vi "Actor Core.vi"(8 "error in":errorcluster, 11 "CS++PPGGUI.lvclass":refnum<class "CS++PPGGui.lvclass">) -> (0 "Error Out":errorcluster, 3 "Actor out":refnum<class "Actor.lvclass">)   [LabVIEW 2016, in "CS++PPGGui.lvlib" / "CS++PPGGui.lvclass"]
doc: "(<B>Filename</B>: Actor Framework.lvlib:Actor.lvclass:Actor Core.vi)\n\nReceives messages to the actor, reacts to them, and initiates any error handling that may shut the actor down.\n\nDescendant classes may override this VI to append parallel tasks for the actor to complete while it handles messages. Overrides use the Call Parent Method node."
uses:
  CS++PPGGui.lvclass
  CSPP_Core/Actors/CS++BaseActor/CS++BaseActor.lvclass
  <vilib>/ActorFramework/Actor/Actor.lvclass
  <vilib>/ActorFramework/Stop Msg/Stop Msg.lvclass
  CSPP_Core/Classes/CS++ProcessVariables/PVConnection/PVConnection.lvclass
  <vilib>/ActorFramework/Message Enqueuer/Message Enqueuer.lvclass
  CSPP_Core/Actors/CS++GUIActor/CS++GUIActor.lvclass
  CSPP_Core/Classes/CS++ProcessVariables/ProcessVariable/PV.lvclass
  CSPP_Core/Actors/CS++DeviceGUIActor/CS++DeviceGUIActor.lvclass
  CSPP_Core/Libraries/Utilities/CS++Utilities.lvlib
  C:/User/Brand/LVP/CSPP-Dev/Packages/CSPP_Core/Actors/CS++DeviceGUIActor/CS++DeviceGUIActor.lvclass
  C:/User/Brand/LVP/CSPP-Dev/Packages/CSPP_Core/Actors/CS++GUIActor/CS++GUIActor.lvclass
  C:/User/Brand/LVP/CSPP-Dev/Packages/CSPP_Core/Actors/CS++BaseActor/CS++BaseActor.lvclass
  C:/Program Files (x86)/National Instruments/LabVIEW 2016/vi.lib/ActorFramework/Actor/Actor.lvclass
panel:
  in  "Tab Control":enum32{"Info", "Control"}(tab)
  out "Last Update":timestamp
  out "Associated Device Actor":string
  out "Resource Name":string
  out "Self-Test Result Message":string
  out "Self-Test Result Code":i32
  out "Firmware Revision":string
  out "Driver Revision":string
  in  "Output":i32(listbox)
  in  "Ext Trig Button":bool
  in  "Abort Button":bool
  in  "Start Single Button":bool
  out "Status String":string
  in  "Pattern2FPGA Button":bool
  in  "Save Button":bool
  in  "Load Button":bool
  out "Error String":string
  in  "Stop Button":bool
  in  "Start Button":bool
  in  "Timing":i32(listbox)
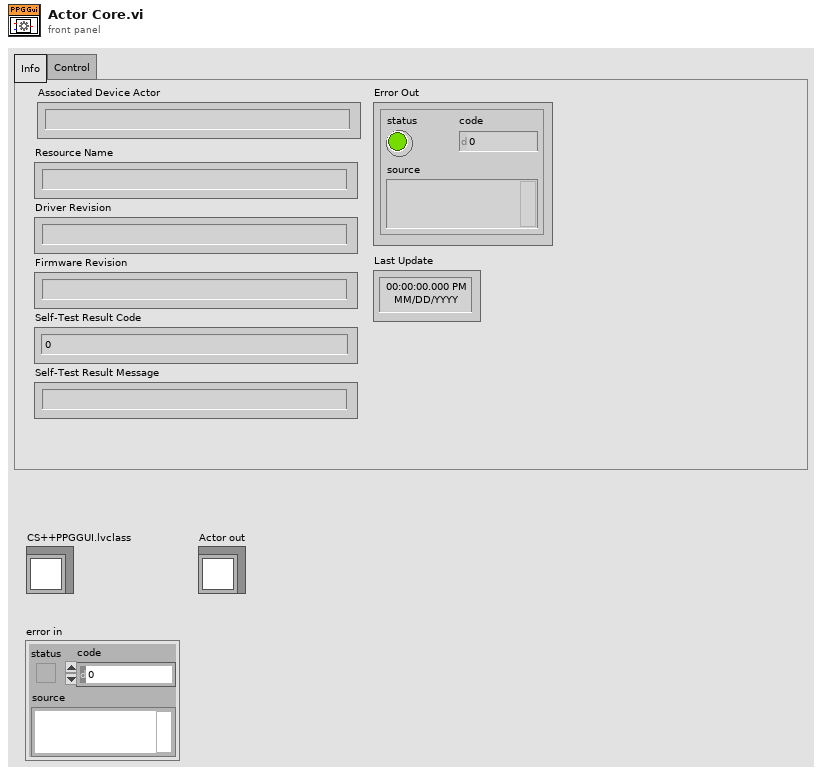
[diagram p1: front panel]
types:
  T1 = enum32{"Invalid", "Standard", "Closed", "Hidden", "Minimized", "Maximized"}
  T2 = enum16{"open", "replace", "create", "open or create", "replace or create", "replace or create with confirmation"}
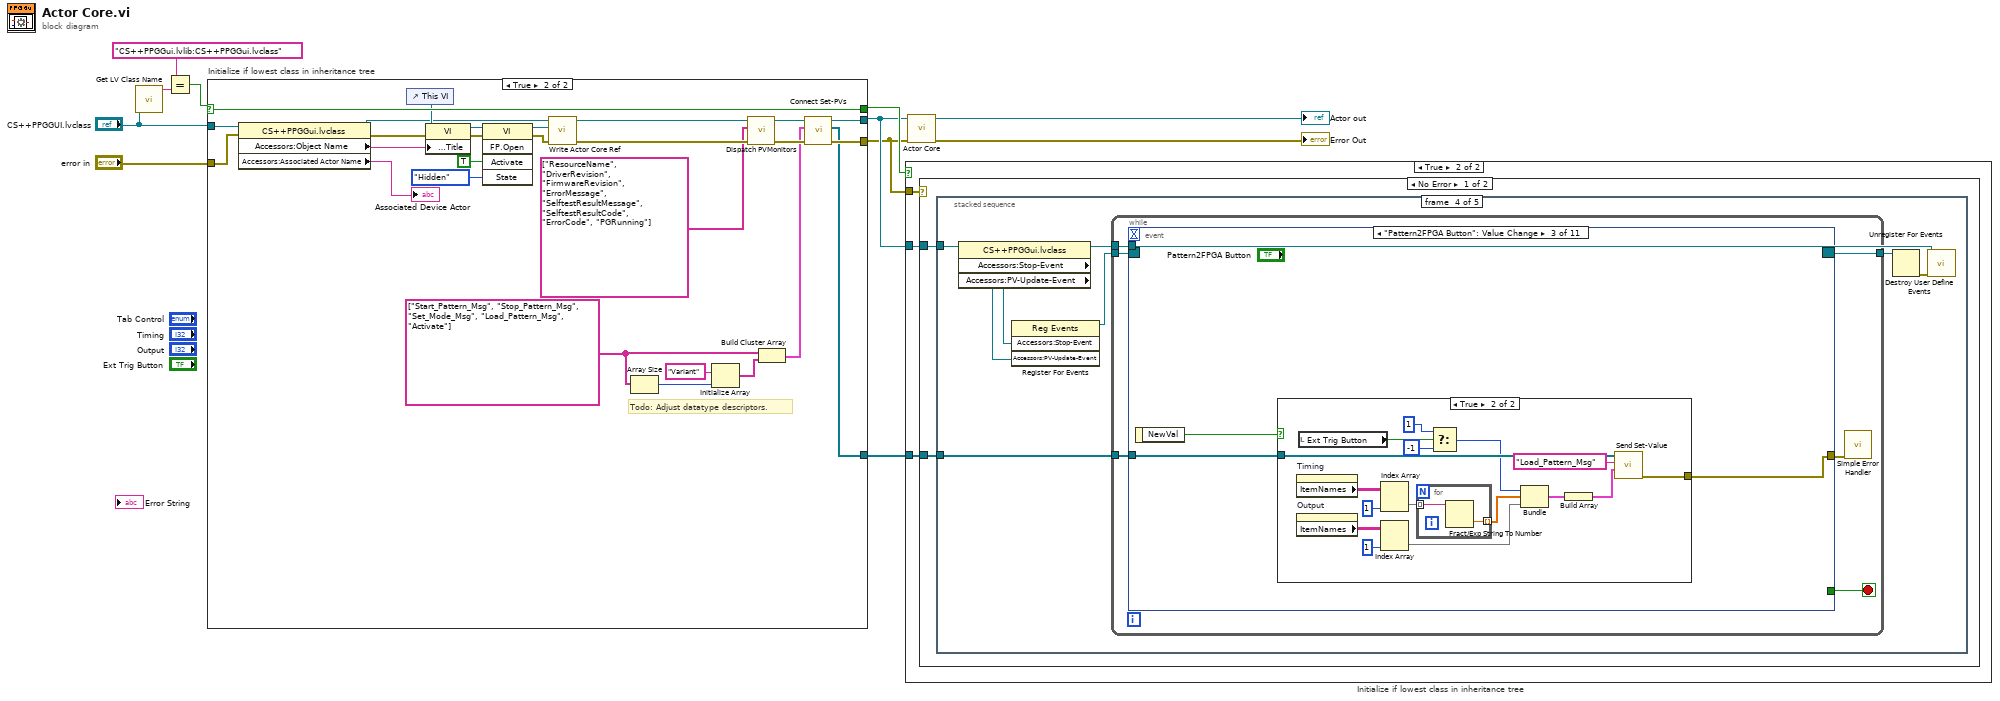
[diagram p0: block diagram]
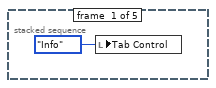
[diagram p4: hidden frame]
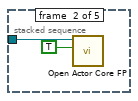
[diagram p5: hidden frame]
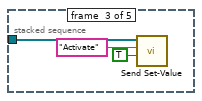
[diagram p6: hidden frame]
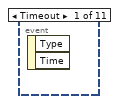
[diagram p7: hidden frame]
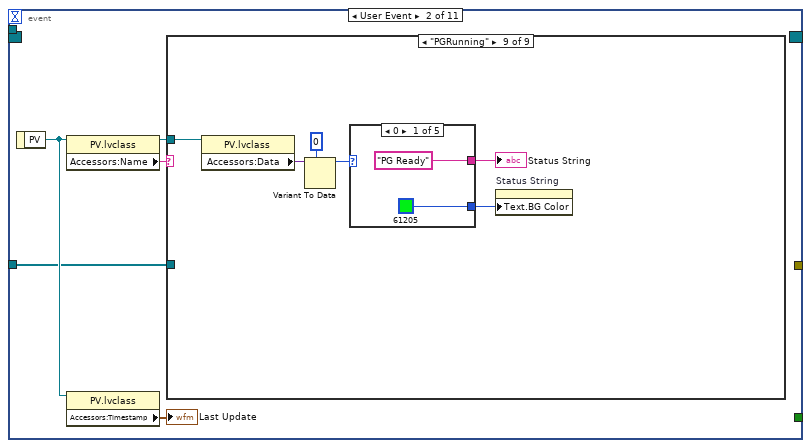
[diagram p8: hidden frame]
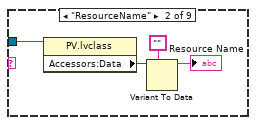
[diagram p10: hidden frame]
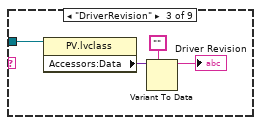
[diagram p11: hidden frame]
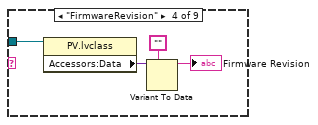
[diagram p12: hidden frame]
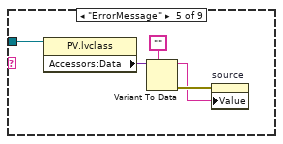
[diagram p13: hidden frame]
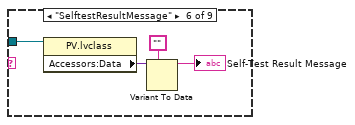
[diagram p14: hidden frame]
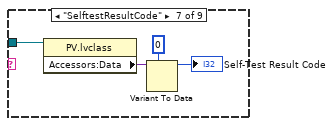
[diagram p15: hidden frame]
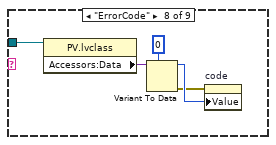
[diagram p16: hidden frame]
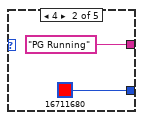
[diagram p17: hidden frame]
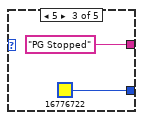
[diagram p18: hidden frame]
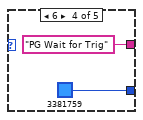
[diagram p19: hidden frame]
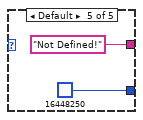
[diagram p20: hidden frame]
diagram:
  n1 = call <vilib>:"Get LV Class Name.vi"("object"="CS++PPGGUI.lvclass") -> ("class name"=w11:string)  [unwired: 9 in, 1 out]
  n2 = Equal?(x="CS++PPGGui.lvlib:CS++PPGGui.lvclass" ("class name"), y=w11) -> (x = y?=w9:bool)
  n3 = case "Initialize if lowest class in inheritance tree" shown="True" w9 {
    selector: w9 -> [w12 w41]
    tunnel: [w13 w24] -> w6
    tunnel: "error in" -> [w13 w28]
    tunnel: [w14 w25] -> w7
    tunnel: "CS++PPGGUI.lvclass" -> [w14 w29]
    tunnel: [w12 w41] -> w8
    tunnel: [_ w22] -> w5
    frame False {
    }
    frame True {
      w21 = string[] ["Start_Pattern_Msg", "Stop_Pattern_Msg", "Set_Mode_Msg", "Load_Pattern_Msg", "Activate"]
      # "Todo: Adjust datatype descriptors."
      n4 = property class="CS++PPGGui.lvclass"(reference=w29, error in=w28) -> (reference out=w33:refnum<class "CS++PPGGui.lvclass">, error out=w27:errorcluster, "Accessors:Object Name"=w32:string, "Accessors:Associated Actor Name"=→"Associated Device Actor":string)
      n5 = control-ref of="This VI"() -> (w36:refnum<vi>)
      n6 = property class="VI"(reference=w36, error in=w27, "Front Panel.Title"=w32) -> (reference out=w35:refnum<vi>, error out=w34:errorcluster)
      n7 = invoke class="VI" method="FP.Open"(reference=w35, error in=w34, "Activate"=TRUE ("Activate?"), "State"=T1."Hidden") -> (reference out=w38:refnum<vi>, error out=w37:errorcluster)  [unwired: 1 in, 3 out]
      n8 = call "Write Actor Core Ref.vi"("error in (no error)"=w37, "Actor Core Ref"=w38, "CS++BaseActor in"=w33) -> ("error out"=w30:errorcluster, "CS++BaseActor out"=w31:refnum<class "CS++PPGGui.lvclass">)  [unwired: 7 in]
      n9 = Array Size(array=w21) -> (size(s)=w20:i32)
      n10 = Initialize Array("Variant", w20) -> (w17:string[])
      n11 = call "Dispatch PVMonitors.vi"("Error In"=w30, "PV Names (empty)"=string[] ["ResourceName", "DriverRevision", "FirmwareRevision", "ErrorMessage", "SelftestResultMessage", "SelftestResultCode", "ErrorCode", "PGRunning"], "CS++GUIActor in"=w31) -> ("Error Out"=w23:errorcluster, "CS++GUIActor out"=w26:refnum<class "CS++PPGGui.lvclass">)  [unwired: 7 in]
      n12 = Build Cluster Array(w21, w17) -> (w18:cluster{string, string}[])
      n13 = call "Connect Set-PVs.vi"("Error In"=w23, "Set-Messages"=w18, "CS++GUIActor in"=w26) -> ("Error Out"=w24:errorcluster, "PVConnections"=w22:refnum<class "PVConnection.lvclass">[], "CS++GUIActor out"=w25:refnum<class "CS++PPGGui.lvclass">)  [unwired: 6 in]
    }
  }
  n14 = case "Initialize if lowest class in inheritance tree" shown="True" w8 {
    tunnel: w6 -> [_ w44]
    tunnel: w7 -> [_ w43]
    tunnel: w5 -> [_ w42]
    frame False {
    }
    frame True {
      n15 = case shown="No Error" w44 {
        tunnel: w43 -> [w46 _]
        tunnel: w42 -> [w45 _]
        frame No Error {
          n16 = stacked-sequence {
            tunnel: w46 -> [_ w48 _ w58 w271]
            tunnel: w45 -> [_ _ w50 w53 w269]
            frame #0 {
              n17 = local write "Tab Control"(enum32{"Info", "Control"}."Info" ("Tab Control")) -> ()
            }
            frame #1 {
              n18 = call "Open Actor Core FP.vi"("Open FP (F)"=TRUE, "CS++BaseActor in"=w48) -> ()  [unwired: 8 in, 2 out]
            }
            frame #2 {
              n19 = call "Send Set-Value.vi"("Data"=TRUE, "PVName"="Activate", "PVConnections"=w50) -> ()  [unwired: 7 in, 2 out]
            }
            frame #3 {
              n20 = property class="CS++PPGGui.lvclass"(reference=w58) -> (reference out=w57:refnum<class "CS++PPGGui.lvclass">, "Accessors:Stop-Event"=w55:refnum<user-event>, "Accessors:PV-Update-Event"=w54:refnum<user-event>)  [unwired: 1 in, 1 out]
              n21 = register-events(w55, w54) -> (reference out=w56:refnum<event-registration>)  [unwired: 2 in, 1 out]
              n22 = while {
                tunnel: w56 -> [w66]
                tunnel: w57 -> [w65]
                tunnel: [w63] -> w60
                tunnel: w53 -> [w61]
                stop <- w64 stop-if-true
                n23 = event shown="[2] \"Pattern2FPGA Button\": Value Change" {
                  selector: w66 -> [_ _ _ _ _ _ _ _ _ _ _]
                  dyn-events: [_ _ _ _ _ _ _ _ _ _ _] -> w63
                  timeout: _ -> [_ _ _ _ _ _ _ _ _ _ _]
                  tunnel: w65 -> [_ _ _ _ _ _ _ w188 w225 w258 w264]
                  tunnel: [_ _ _ _ _ _ _ _ _ TRUE ("Stop") TRUE ("Stop")] -> w64
                  tunnel: [_ _ w118 w139 w156 w173 w180 w189 w222 _ errorcluster {"status"=FALSE, "code"=0, "source"=""} ("error IO")] -> w62
                  tunnel: w61 -> [_ w68 w119 w140 w157 w174 w181 _ _ _ _]
                  event Timeout {
                    n24 = event-data() -> ()  [unwired: 1 in, 2 out]
                  }
                  event User Event {
                    n25 = event-data() -> ("PV"=w70:refnum<class "PV.lvclass">)  [unwired: 1 in]
                    n26 = property class="PV.lvclass"(reference=w70) -> (reference out=w71:refnum<class "PV.lvclass">, "Accessors:Name"=w67:string)  [unwired: 1 in, 1 out]
                    n27 = property class="PV.lvclass"(reference=w70) -> ("Accessors:Timestamp"=→"Last Update":timestamp)  [unwired: 1 in, 2 out]
                    n28 = case shown="\"PGRunning\"" w67 {
                      tunnel: w71 -> [_ w73 w77 w81 w86 w90 w94 w99 w105]
                      tunnel: w68 -> [_ _ _ _ _ _ _ _ _]
                      frame Default {
                      }
                      frame "ResourceName" {
                        n29 = property class="PV.lvclass"(reference=w73) -> ("Accessors:Data"=w75:variant)  [unwired: 1 in, 2 out]
                        n30 = Variant To Data(type="", Variant=w75) -> (data=→"Resource Name":string)  [unwired: 1 in, 1 out]
                      }
                      frame "DriverRevision" {
                        n31 = property class="PV.lvclass"(reference=w77) -> ("Accessors:Data"=w79:variant)  [unwired: 1 in, 2 out]
                        n32 = Variant To Data(type="", Variant=w79) -> (data=→"Driver Revision":string)  [unwired: 1 in, 1 out]
                      }
                      frame "FirmwareRevision" {
                        n33 = property class="PV.lvclass"(reference=w81) -> ("Accessors:Data"=w83:variant)  [unwired: 1 in, 2 out]
                        n34 = Variant To Data(type="", Variant=w83) -> (data=→"Firmware Revision":string)  [unwired: 1 in, 1 out]
                      }
                      frame "ErrorMessage" {
                        n35 = property class="PV.lvclass"(reference=w86) -> ("Accessors:Data"=w88:variant)  [unwired: 1 in, 2 out]
                        n36 = Variant To Data(type="", Variant=w88) -> (data=w84:string, error out=w85:errorcluster)  [unwired: 1 in]
                        n37 = property on="source" class="Str"(error in=w85, "Value"=w84) -> ()  [unwired: 1 in, 2 out]
                      }
                      frame "SelftestResultMessage" {
                        n38 = property class="PV.lvclass"(reference=w90) -> ("Accessors:Data"=w92:variant)  [unwired: 1 in, 2 out]
                        n39 = Variant To Data(type="", Variant=w92) -> (data=→"Self-Test Result Message":string)  [unwired: 1 in, 1 out]
                      }
                      frame "SelftestResultCode" {
                        n40 = property class="PV.lvclass"(reference=w94) -> ("Accessors:Data"=w96:variant)  [unwired: 1 in, 2 out]
                        n41 = Variant To Data(type=0, Variant=w96) -> (data=→"Self-Test Result Code":i32)  [unwired: 1 in, 1 out]
                      }
                      frame "ErrorCode" {
                        n42 = property class="PV.lvclass"(reference=w99) -> ("Accessors:Data"=w101:variant)  [unwired: 1 in, 2 out]
                        n43 = Variant To Data(type=0, Variant=w101) -> (data=w98:i32, error out=w97:errorcluster)  [unwired: 1 in]
                        n44 = property on="code" class="DigNum (strict)"(error in=w97, "Value"=w98) -> ()  [unwired: 1 in, 2 out]
                      }
                      frame "PGRunning" {
                        n45 = property class="PV.lvclass"(reference=w105) -> ("Accessors:Data"=w107:variant)  [unwired: 1 in, 2 out]
                        n46 = Variant To Data(type=0, Variant=w107) -> (data=w104:i32)  [unwired: 1 in, 1 out]
                        n47 = case shown="0" w104 {
                          tunnel: ["PG Ready" "PG Running" "PG Stopped" "PG Wait for Trig" "Not Defined!"] -> w103
                          tunnel: [u32 61205 u32 16711680 u32 16776722 u32 3381759 u32 16448250] -> w102
                          frame 0 {
                          }
                          frame 4 {
                          }
                          frame 5 {
                          }
                          frame 6 {
                          }
                          frame Default {
                          }
                        }
                        "Status String" <- w103
                        n48 = property on="Status String" class="Str"("Text.BG Color"=w102) -> ()  [unwired: 2 in, 2 out]
                      }
                    }
                  }
                  event "Pattern2FPGA Button": Value Change {
                    n49 = event-data() -> ("NewVal"=w120:bool)  [unwired: 1 in]
                    n50 = case shown="True" w120 {
                      tunnel: w119 -> [_ w136]
                      tunnel: [_ w134] -> w118
                      frame False {
                      }
                      frame True {
                        n51 = property on="Timing" class="MCListbox (strict)"() -> ("ItemNames"=w133:string[][])  [unwired: 2 in, 2 out]
                        n52 = property on="Output" class="MCListbox (strict)"() -> ("ItemNames"=w130:string[][])  [unwired: 2 in, 2 out]
                        n53 = local read "Ext Trig Button"() -> (w128:bool)
                        n54 = Index Array(array=w133, index (col)=1 ("disabled index (col)")) -> (element=w122:string[])  [unwired: 1 in]
                        n55 = Index Array(array=w130, index (col)=1 ("disabled index (col)")) -> (element=w129:string[])  [unwired: 1 in]
                        n56 = for {
                          tunnel: w122 -> [w138] mode=indexing
                          tunnel: [w137] -> w121 mode=indexing
                          n57 = Fract/Exp String To Number(string=w138) -> (number=w137:dbl)  [unwired: 3 in, 1 out]
                        }
                        n58 = Select(t=1, s=w128, f=-1) -> (s? t:f=w127:i32)
                        n59 = Bundle(w127, w121, "ItemNames"=w129) -> (w124:cluster{i32, dbl[], "ItemNames":string[]})  [unwired: 1 in]
                        n60 = Build Array(w124) -> (w123:cluster{i32, dbl[], "ItemNames":string[]}[])
                        n61 = call "Send Set-Value.vi"("Data"=w123, "PVName"="Load_Pattern_Msg", "PVConnections"=w136) -> ("error out"=w134:errorcluster)  [unwired: 7 in, 1 out]
                      }
                    }
                  }
                  event "Start Button": Value Change {
                    n62 = event-data() -> ("NewVal"=w141:bool)  [unwired: 1 in]
                    n63 = case shown="True" w141 {
                      tunnel: w140 -> [_ w144]
                      tunnel: [_ w145] -> w139
                      frame False {
                      }
                      frame True {
                        n64 = flat-sequence {
                          tunnel: w144 -> [w150]
                          tunnel: [w150] -> w143
                          tunnel: [w149] -> w142
                          tunnel: [w155] -> w145
                          tunnel: w143 -> [w153]
                          tunnel: w142 -> [w152]
                          frame #0 {
                            n65 = Wait (ms)(milliseconds to wait=u32 20) -> ()  [unwired: 1 out]
                            n66 = call "Send Set-Value.vi"("Data"=u8 1, "PVName"="Set_Mode_Msg", "PVConnections"=w150) -> ("error out"=w149:errorcluster)  [unwired: 7 in, 1 out]
                          }
                          frame #1 {
                            n67 = call "Send Set-Value.vi"("error in (no error)"=w152, "Data"=0, "PVName"="Start_Pattern_Msg", "PVConnections"=w153) -> ("error out"=w155:errorcluster)  [unwired: 6 in, 1 out]
                          }
                        }
                      }
                    }
                  }
                  event "Start Single Button": Value Change {
                    n68 = event-data() -> ("NewVal"=w158:bool)  [unwired: 1 in]
                    n69 = case shown="True" w158 {
                      tunnel: w157 -> [_ w160]
                      tunnel: [_ w159] -> w156
                      frame False {
                      }
                      frame True {
                        n70 = flat-sequence {
                          tunnel: w160 -> [w167]
                          tunnel: [w167] -> w162
                          tunnel: [w166] -> w161
                          tunnel: [w172] -> w159
                          tunnel: w162 -> [w170]
                          tunnel: w161 -> [w169]
                          frame #0 {
                            n71 = Wait (ms)(milliseconds to wait=u32 20) -> ()  [unwired: 1 out]
                            n72 = call "Send Set-Value.vi"("Data"=u8 0, "PVName"="Set_Mode_Msg", "PVConnections"=w167) -> ("error out"=w166:errorcluster)  [unwired: 7 in, 1 out]
                          }
                          frame #1 {
                            n73 = call "Send Set-Value.vi"("error in (no error)"=w169, "Data"=0, "PVName"="Start_Pattern_Msg", "PVConnections"=w170) -> ("error out"=w172:errorcluster)  [unwired: 6 in, 1 out]
                          }
                        }
                      }
                    }
                  }
                  event "Stop Button": Value Change {
                    n74 = event-data() -> ("NewVal"=w175:bool)  [unwired: 1 in]
                    n75 = case shown="True" w175 {
                      tunnel: w174 -> [_ w179]
                      tunnel: [_ w177] -> w173
                      frame False {
                      }
                      frame True {
                        n76 = call "Send Msg Trigger.vi"("Trigger Msg (F)"=TRUE, "PVName"="Stop_Pattern_Msg", "PVConnections"=w179) -> ("error out"=w177:errorcluster)  [unwired: 7 in, 1 out]
                      }
                    }
                  }
                  event "Abort Button": Value Change {
                    n77 = event-data() -> ("NewVal"=w182:bool)  [unwired: 1 in]
                    n78 = case shown="True" w182 {
                      tunnel: w181 -> [_ w186]
                      tunnel: [_ w184] -> w180
                      frame False {
                      }
                      frame True {
                        n79 = call "Send Msg Trigger.vi"("Trigger Msg (F)"=TRUE, "PVName"="Stop_Pattern_Msg", "PVConnections"=w186) -> ("error out"=w184:errorcluster)  [unwired: 7 in, 1 out]
                      }
                    }
                  }
                  event "Save Button": Value Change {
                    n80 = event-data() -> ("NewVal"=w190:bool)  [unwired: 1 in]
                    n81 = property class="CS++PPGGui.lvclass"(reference=w188) -> ("Accessors:Object Name"=w187:string)  [unwired: 1 in, 2 out]
                    n82 = case shown="True" w190 {
                      tunnel: [_ w198] -> w189
                      tunnel: w187 -> [_ w194]
                      frame False {
                      }
                      frame True {
                        n83 = property on="Timing" class="MCListbox (strict)"() -> ("ItemNames"=w208:string[][])  [unwired: 2 in, 2 out]
                        n84 = property on="Output" class="MCListbox (strict)"() -> ("ItemNames"=w207:string[][])  [unwired: 2 in, 2 out]
                        n85 = for {
                          tunnel: w208 -> [w221] mode=indexing
                          tunnel: [w219] -> w204 mode=indexing
                          n86 = call "String Array 2 String.vi"("Substrings"=w221, "Delimiter (\",\")"="|") -> ("String"=w219:string)
                        }
                        n87 = for {
                          tunnel: w207 -> [w218] mode=indexing
                          tunnel: [w216] -> w205 mode=indexing
                          n88 = call "String Array 2 String.vi"("Substrings"=w218, "Delimiter (\",\")"="|") -> ("String"=w216:string)
                        }
                        n89 = call "String Array 2 String.vi"("Substrings"=w204, "Delimiter (\",\")"="/") -> ("String"=w203:string)
                        n90 = call "String Array 2 String.vi"("Substrings"=w205, "Delimiter (\",\")"="/") -> ("String"=w202:string)
                        n91 = Build Array(w203, w202) -> (w200:string[])
                        n92 = call "String Array 2 String.vi"("Substrings"=w200, "Delimiter (\",\")"="\\") -> ("String"=w199:string)
                        n93 = Open/Create/Replace File(operation (0:open)=T2."replace or create with confirmation", access (0:read/write)=enum16{"read/write", "read-only", "write-only"}."write-only") -> (refnum out=w213:refnum<file>, error out=w212:errorcluster)  [unwired: 4 in, 1 out]
                        n94 = Write to Text File(file (use dialog)=w213, text=w199, error in=w212) -> (refnum out=w215:refnum<file>, error out=w214:errorcluster)  [unwired: 1 in, 1 out]
                        n95 = control-ref of="This VI"() -> (w196:refnum<vi>)
                        n96 = Close File(refnum=w215, error in=w214) -> (path=w192:path, error out=w195:errorcluster)
                        n97 = Strip Path(path=w192) -> (name=w191:string)  [unwired: 1 out]
                        n98 = Concatenate Strings(w194, " - " ("string"), w191) -> (w197:string)
                        n99 = property class="VI"(reference=w196, error in=w195, "Front Panel.Title"=w197) -> (error out=w198:errorcluster)  [unwired: 1 out]
                      }
                    }
                  }
                  event "Load Button": Value Change {
                    n100 = event-data() -> ("NewVal"=w224:bool)  [unwired: 1 in]
                    n101 = property class="CS++PPGGui.lvclass"(reference=w225) -> ("Accessors:Object Name"=w223:string)  [unwired: 1 in, 2 out]
                    n102 = case shown="True" w224 {
                      tunnel: w223 -> [_ w235]
                      tunnel: [_ w234] -> w222
                      frame False {
                      }
                      frame True {
                        w240 = "/"
                        n103 = Open/Create/Replace File(access (0:read/write)=enum16{"read/write", "read-only", "write-only"}."read-only") -> (refnum out=w248:refnum<file>, error out=w247:errorcluster)  [unwired: 5 in, 1 out]
                        n104 = Read from Text File(file (use dialog)=w248, error in=w247) -> (refnum out=w250:refnum<file>, text=w246:string, error out=w249:errorcluster)  [unwired: 2 in, 1 out]
                        n105 = call "String 2 String Array.vi"("String"=w246, "Delimiter (\",\")"="\\") -> ("Substrings"=w243:string[])
                        n106 = Close File(refnum=w250, error in=w249) -> (path=w233:path)  [unwired: 1 out]
                        n107 = Index Array(array=w243) -> (element #1=w242:string, element #2=w241:string)  [unwired: 2 in]
                        n108 = call "String 2 String Array.vi"("String"=w242, "Delimiter (\",\")"=w240) -> ("Substrings"=w232:string[])
                        n109 = call "String 2 String Array.vi"("String"=w241, "Delimiter (\",\")"=w240) -> ("Substrings"=w230:string[])
                        n110 = for {
                          tunnel: w232 -> [w255] mode=indexing
                          tunnel: [w254] -> w231 mode=indexing
                          n111 = call "String 2 String Array.vi"("String"=w255, "Delimiter (\",\")"="|") -> ("Substrings"=w254:string[])
                        }
                        n112 = for {
                          tunnel: w230 -> [w252] mode=indexing
                          tunnel: [w251] -> w229 mode=indexing
                          n113 = call "String 2 String Array.vi"("String"=w252, "Delimiter (\",\")"="|") -> ("Substrings"=w251:string[])
                        }
                        n114 = property on="Timing" class="MCListbox (strict)"("ItemNames"=w231) -> (error out=w228:errorcluster)  [unwired: 2 in, 1 out]
                        n115 = property on="Output" class="MCListbox (strict)"("ItemNames"=w229) -> (error out=w227:errorcluster)  [unwired: 2 in, 1 out]
                        n116 = Strip Path(path=w233) -> (name=w239:string)  [unwired: 1 out]
                        n117 = Merge Errors(w228, w227) -> (w226:errorcluster)
                        n118 = Concatenate Strings(w235, " - " ("string"), w239) -> (w236:string)
                        n119 = control-ref of="This VI"() -> (w237:refnum<vi>)
                        n120 = property class="VI"(reference=w237, error in=w226, "Front Panel.Title"=w236) -> (error out=w234:errorcluster)  [unwired: 1 out]
                      }
                    }
                  }
                  event Panel Close? {
                    n121 = event-data() -> ()  [unwired: 1 in, 1 out]
                    n122 = call <vilib>:"Read Self Enqueuer.vi"("Actor"=w258) -> ("Self Enqueuer"=w260:refnum<class "Message Enqueuer.lvclass">)  [unwired: 10 in]
                    n123 = call <vilib>:"Send Normal Stop.vi"("Message Enqueuer"=w260) -> ("error out"=w259:errorcluster)  [unwired: 10 in]
                    n124 = call <vilib>:"Simple Error Handler.vi"("error in (no error)"=w259) -> ()  [unwired: 4 in, 5 out]
                    n125 = event-data("Discard?"=TRUE) -> ()  [unwired: 1 in, 1 out]
                  }
                  event User Event {
                    n126 = event-data() -> ()  [unwired: 1 in, 5 out]
                    n127 = call <vilib>:"Read Self Enqueuer.vi"("Actor"=w264) -> ("Self Enqueuer"=w266:refnum<class "Message Enqueuer.lvclass">)  [unwired: 10 in]
                    n128 = call <vilib>:"Send Normal Stop.vi"("Message Enqueuer"=w266) -> ("error out"=w265:errorcluster)  [unwired: 10 in]
                    n129 = call <vilib>:"Simple Error Handler.vi"("error in (no error)"=w265) -> ()  [unwired: 4 in, 5 out]
                  }
                }
                n130 = call <vilib>:"Simple Error Handler.vi"("error in (no error)"=w62) -> ()  [unwired: 4 in, 5 out]
              }
              n131 = Unregister For Events(event registration refnum=w60) -> (error out=w59:errorcluster)  [unwired: 1 in]
              n132 = call-dynamic "Destroy User Define Events.vi"("error in (no error)"=w59, "CS++GUIActor in"=w57) -> ()  [unwired: 8 in, 2 out]
            }
            frame #4 {
              # "ToDo: This destroys the complete device object.\nMaybe someone only wants to close the GUI. \nBut in this case one should also be able to only \nopen the GUI without starting a second Proxy which\nwill not work (--> Object Manager)"
              n133 = for {
                tunnel: w269 -> [w281] mode=indexing
                n134 = call "Disconnect.vi"("PVConnection in"=w281) -> ()  [unwired: 9 in, 2 out]
              }
              n135 = call "Open Actor Core FP.vi"("Open FP (F)"=FALSE, "CS++BaseActor in"=w271) -> ("error out"=w267:errorcluster, "CS++BaseActor out"=w268:refnum<class "CS++PPGGui.lvclass">)  [unwired: 8 in]
              n136 = disable-structure shown="Enabled" {
                disable-tunnel: w268 -> [w276 _]
                disable-tunnel: w267 -> [w274 _]
                frame Enabled {
                  n137 = property class="CS++PPGGui.lvclass"(reference=w276, error in=w274) -> (error out=w275:errorcluster, "Accessors:Associated Proxy Actor Enqueuer"=w273:refnum<class "Message Enqueuer.lvclass">)  [unwired: 1 out]
                  n138 = call <vilib>:"Equals Not A Refnum.vi"("Message Enqueuer"=w273) -> ("Not a refnum?"=w272:bool)  [unwired: 10 in]
                  n139 = case shown="False" w272 {
                    tunnel: [w279 w280] -> _
                    tunnel: w273 -> [w278 _]
                    tunnel: w275 -> [w277 w280]
                    frame False {
                      n140 = call <vilib>:"Send Normal Stop.vi"("error in (no error)"=w277, "Message Enqueuer"=w278) -> ("error out"=w279:errorcluster)  [unwired: 9 in]
                    }
                    frame True {
                    }
                  }
                }
                frame Disabled {
                }
              }
            }
          }
        }
        frame Error {
        }
      }
    }
  }
  n141 = call-parent "Actor Core.vi"("error in"=w6, "CS++DeviceGUIActor.lvclass"=w7) -> ("Error Out"=→"Error Out":errorcluster, "Actor out"=→"Actor out":refnum<class "Actor.lvclass">)  [unwired: 8 in]
